vi "main.vi"() -> ()   [LabVIEW 2016]
uses:
  enum_setting_states.ctl
  <vilib>/Instr/_visa.llb/VISA Configure Serial Port (Instr).vi
  global.vi
panel:
  out "Tab Control":enum32{"Settings", "Data"}(tab)
  in  "Boolean":bool
  in  "4th":dbl=4.0 min=1.0 step=1.0 format="%#_3g"
  in  "3rd":dbl=3.0 min=1.0 step=1.0 format="%#_3g"
  in  "2nd":dbl=2.0 min=1.0 step=1.0 format="%#_3g"
  in  "1st":dbl=1.0 min=1.0 step=1.0 format="%#_3g"
  in  "START":bool
  in  "SET":bool
  in  "Flow control (None)":u16(ring) items=["None", "XON/XOFF", "RTS/CTS", "XON/XOFF & RTS/CTS", "DTR/DSR", "XON/XOFF & DTR/DSR"]
  in  "Parity (None)":enum16{"None", "Odd", "Even", "Mark", "Space"}(ring)
  in  "Stop bits (1)":u16(ring)=10 items=["1.0"=10, "1.5"=15, "2.0"=20]
  in  "Data bits (8)":u16=8 min=5 max=8 step=1
  in  "Baud rate (57600)":u32=57600
  in  "VISA resource name":refnum<visa-resource-name>="COM5"
  out "read buffer":string
  in  "Charge current":enum8{"0.25C", "0.5C", "1C"}(ring)=enum."0.5C"
  in  "Discharge current":enum8{"0.25C", "0.5C", "1C"}(ring)=enum."1C"
  in  "Number of cells":enum8{"", "1", "2", "3", "4"}(ring)=enum."1"
  in  "Options":T1(ring)=enum."Predischarge->Charge->Discharge->Postcharge"
  in  "Project Name":string="Test"
  out "Cell number":string
  out "State":string
  out "Path":path
  in  "stop":bool
  out "TEMP":dbl caption="Current Temperature\n(Celsius)"
  out "CURRENT":dbl caption="Current Temperature\n(Celsius)"
  out "VOLTAGE":dbl caption="Current Temperature\n(Celsius)"
  in  "next":bool
  out "Countdown":dbl caption="Current Temperature\n(Celsius)"
  out "min":dbl caption="Current Temperature\n(Celsius)"
  out "sec":dbl caption="Current Temperature\n(Celsius)"
  out "CAPACITY":dbl caption="Current Temperature\n(Celsius)"
  out "Voltage":cluster{dbl[], dbl[]}(graph)
  out "Current":cluster{dbl[], dbl[]}(graph)
  out "Temperature":cluster{dbl[], dbl[]}(graph)
  out "Capacity":cluster{dbl[], dbl[]}(graph)
  out "Received data":string
  # "UART configurations"
  # "Test configurations"
  # "Cell order"
  # "Elapsed time"
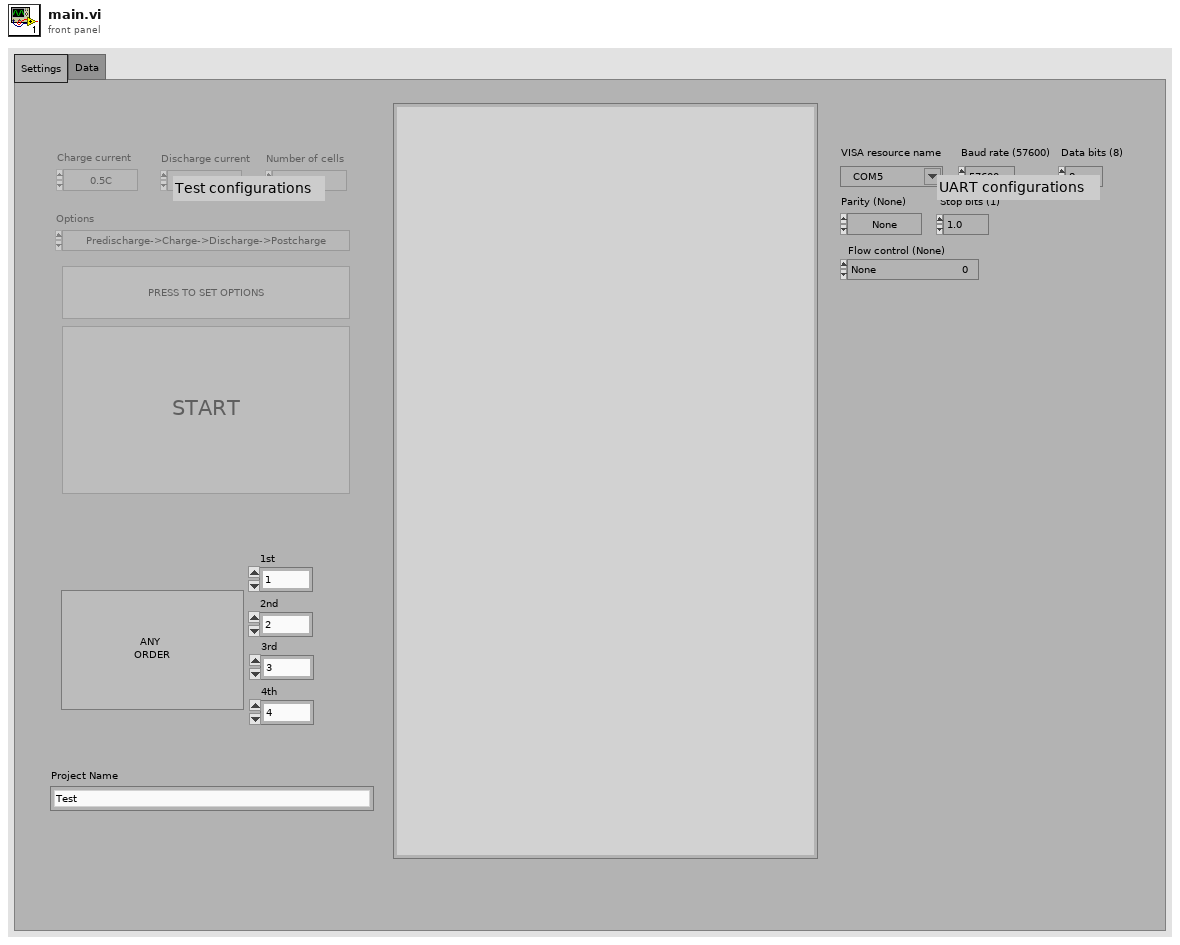
[diagram p1: front panel]
types:
  T1 = enum8{"", "Predischarge->Charge->Discharge->Postcharge", "Charge->Discharge", "Only Charge", "Only Discharge"}
  T2 = enum8{"Enabled", "Disabled", "Disabled and Grayed Out"}
  T3 = typedef "enum_setting_states.ctl" = enum16{"Initialize", "Charge_current", "Discharge_current", "Option", "Num_of_cells", "Start"}
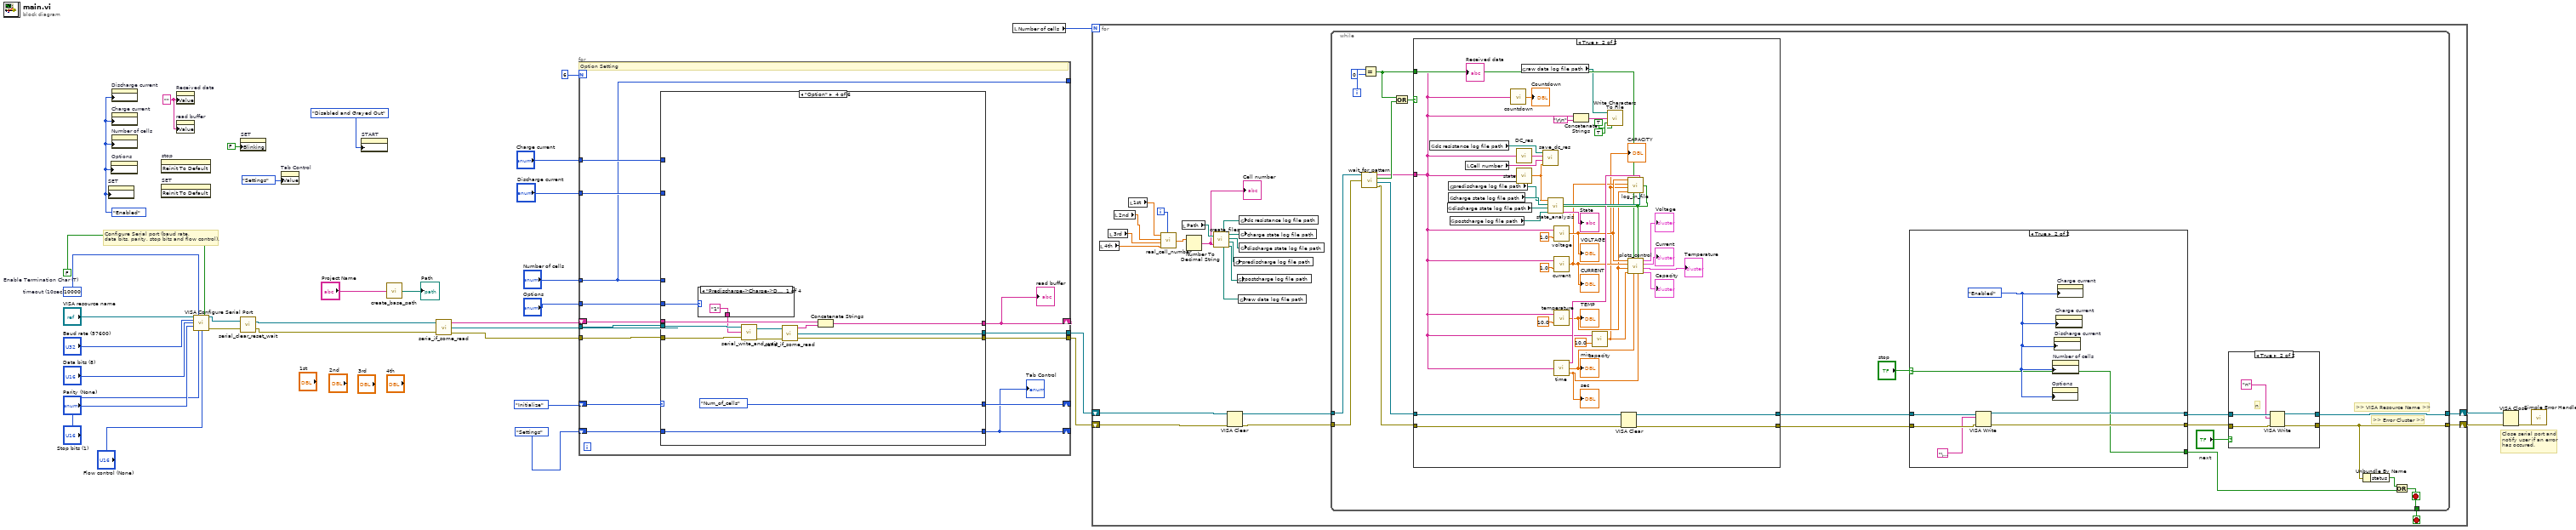
[diagram p0: block diagram]
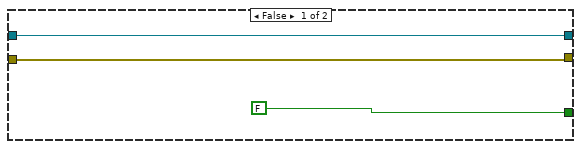
[diagram p4: hidden frame]
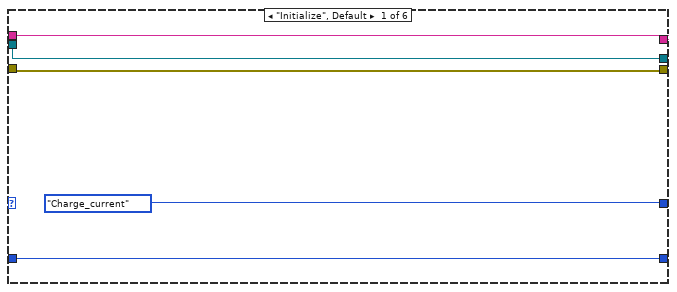
[diagram p5: hidden frame]
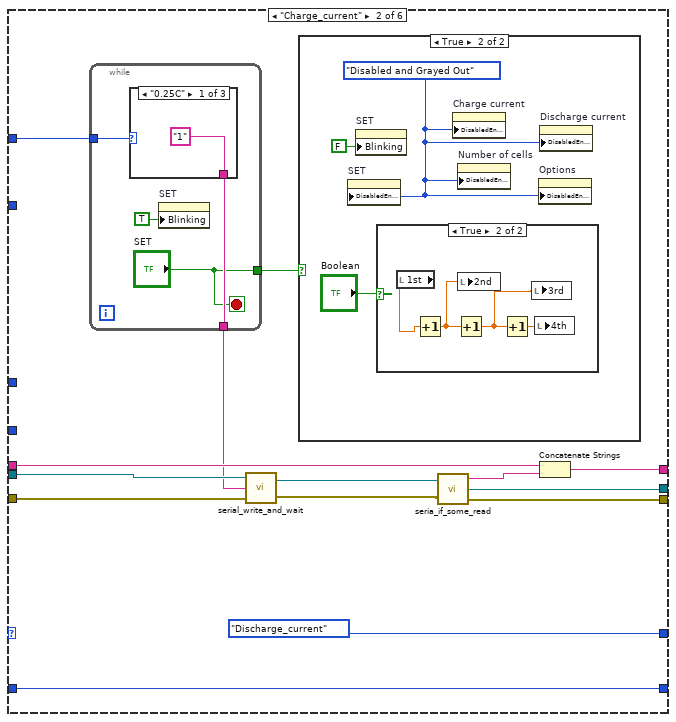
[diagram p6: hidden frame]
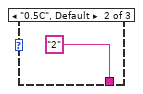
[diagram p9: hidden frame]
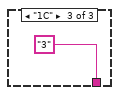
[diagram p10: hidden frame]
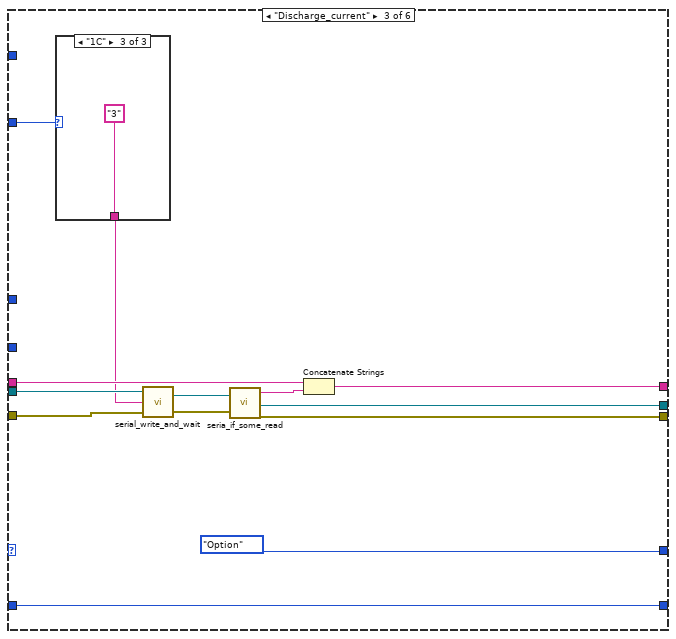
[diagram p11: hidden frame]
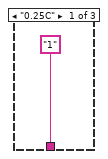
[diagram p12: hidden frame]
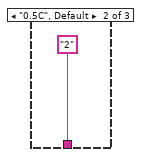
[diagram p13: hidden frame]
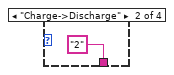
[diagram p14: hidden frame]
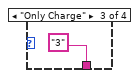
[diagram p15: hidden frame]
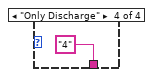
[diagram p16: hidden frame]
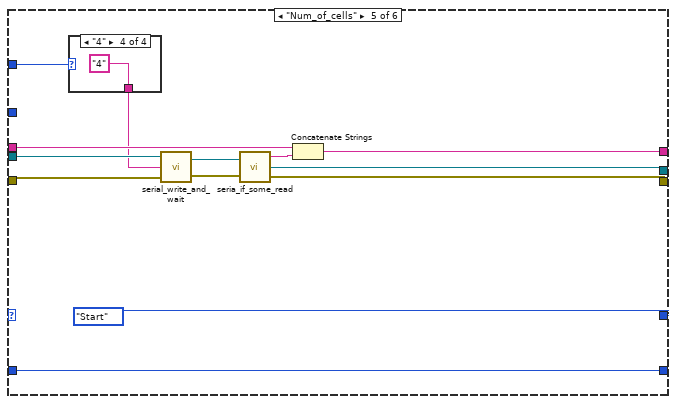
[diagram p17: hidden frame]
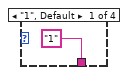
[diagram p18: hidden frame]
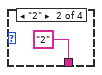
[diagram p19: hidden frame]
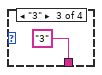
[diagram p20: hidden frame]
diagram:
  w12 = T2."Enabled" ("Disabled")
  w10 = "" ("read buffer")
  w34 = FALSE  # Enable Termination Char (T)
  w35 = u32 10000  # timeout (10sec)
  # "Close serial port and\nnotify user if an error\nhas occured."
  # "Configure Serial port (baud rate,\ndata bits, parity, stop bits and flow control)."
  n1 = property on="SET" class="Bool (strict)"("DisabledEnum"=w12) -> ()  [unwired: 2 in, 2 out]
  n2 = property on="Options" class="Enum (strict)"("DisabledEnum"=w12) -> ()  [unwired: 2 in, 2 out]
  n3 = property on="Discharge current" class="Enum (strict)"("DisabledEnum"=w12) -> ()  [unwired: 2 in, 2 out]
  n4 = property on="Charge current" class="Enum (strict)"("DisabledEnum"=w12) -> ()  [unwired: 2 in, 2 out]
  n5 = property on="Number of cells" class="Enum (strict)"("DisabledEnum"=w12) -> ()  [unwired: 2 in, 2 out]
  n6 = invoke on="stop" class="Bool" method="Reinit To Default"() -> ()  [unwired: 3 in, 3 out]
  n7 = invoke on="SET" class="Bool (strict)" method="Reinit To Default"() -> ()  [unwired: 3 in, 3 out]
  n8 = property on="Received data" class="Str"("Value"=w10) -> ()  [unwired: 2 in, 2 out]
  n9 = property on="read buffer" class="Str"("Value"=w10) -> ()  [unwired: 2 in, 2 out]
  n10 = call-poly "VISA Configure Serial Port"("VISA resource name"="VISA resource name", "timeout (10sec)"=w35, "Enable Termination\nChar (T)"=w34, "baud rate (9600)"="Baud rate (57600)", "data bits (8)"="Data bits (8)", "parity (0:none)"="Parity (None)", "stop bits (10: 1 bit)"="Stop bits (1)", "flow control (0:none)"="Flow control (None)") -> ("VISA resource name out"=w32:refnum<visa-resource-name>, "error out"=w33:errorcluster)  [unwired: 6 in]
  n11 = property on="SET" class="Bool (strict)"("Blinking"=FALSE) -> ()  [unwired: 2 in, 2 out]
  n12 = call "serial_clear_reset_wait.vi"("error in (no error)"=w33, "VISA Refnum in"=w32) -> ("error out"=w17:errorcluster, "VISA Refnum out"=w18:refnum<visa-resource-name>)
  n13 = property on="Tab Control" class="TabCtl (strict)"("Value"=enum32{"Settings", "Data"}."Settings" ("Tab Control")) -> ()  [unwired: 2 in, 2 out]
  n14 = property on="START" class="Bool"("DisabledEnum"=T2."Disabled and Grayed Out" ("Disabled")) -> ()  [unwired: 2 in, 2 out]
  n15 = call "create_base_path.vi"("project name"="Project Name") -> ("base path"=→"Path":path)
  n16 = call "seria_if_some_read.vi"("serial in"=w18, "error in (no error)"=w17) -> ("read buffer"=w8:string, "serial out"=w9:refnum<visa-resource-name>, "error out"=w20:errorcluster)
  n17 = for {
    N: 6 -> [_]
    shift-right: [w38] -> _
    shift-left: enum32{"Settings", "Data"}."Settings" ("Tab Control") -> [w47]
    shift-right: [w46] -> _
    shift-left: enum_setting_states."Initialize" -> [w45]
    tunnel: w9 -> [w43]
    tunnel: [w49] -> w3
    tunnel: w20 -> [w42]
    tunnel: [w48] -> w2
    tunnel: "Charge current" -> [w41]
    shift-right: [w44] -> _
    shift-left: w8 -> [w40]
    tunnel: "Discharge current" -> [w39]
    tunnel: "Number of cells" -> [w36]
    tunnel: "Options" -> [w37]
    tunnel: [w36] -> _
    # "Option Setting"
    n18 = case shown="\"Option\"" w45 {
      tunnel: w43 -> [w53 w66 w90 w103 w123 w140]
      tunnel: w42 -> [w52 w65 w88 w101 w121 w139]
      tunnel: [w51 w63 w93 w110 w126 w145] -> w44
      tunnel: [w53 w56 w84 w105 w117 w134] -> w49
      tunnel: [w52 w55 w83 w104 w116 w133] -> w48
      tunnel: [w50 w60 w91 w107 w124 enum32{"Settings", "Data"}."Data" ("Tab Control")] -> w38
      tunnel: w47 -> [w50 w60 w91 w107 w124 _]
      tunnel: [enum_setting_states."Charge_current" enum_setting_states."Discharge_current" enum_setting_states."Option" enum_setting_states."Num_of_cells" enum_setting_states."Start" enum_setting_states."Start"] -> w46
      tunnel: w40 -> [w51 w64 w94 w111 w127 w144]
      tunnel: w41 -> [_ w67 _ _ _ _]
      tunnel: w39 -> [_ _ w92 _ _ _]
      tunnel: w36 -> [_ _ _ _ w125 _]
      tunnel: w37 -> [_ _ _ w108 _ _]
      frame "Initialize", Default {
      }
      frame "Charge_current" {
        n19 = while {
          tunnel: w67 -> [w79]
          tunnel: [w78] -> w62
          tunnel: ["SET"] -> w61
          stop <- "SET" stop-if-true
          n20 = case shown="\"0.25C\"" w79 {
            tunnel: ["1" ("write buffer") "2" ("write buffer") "3" ("write buffer")] -> w78
            frame "0.25C" {
            }
            frame "0.5C", Default {
            }
            frame "1C" {
            }
          }
          n21 = property on="SET" class="Bool (strict)"("Blinking"=TRUE) -> ()  [unwired: 2 in, 2 out]
        }
        n22 = call "serial_write_and_wait.vi"("error in (no error)"=w65, "write buffer"=w62, "serial in"=w66) -> ("error out"=w58:errorcluster, "serial out"=w59:refnum<visa-resource-name>)
        n23 = case shown="True" w61 {
          frame False {
          }
          frame True {
            w70 = T2."Disabled and Grayed Out" ("Disabled")
            n24 = property on="SET" class="Bool (strict)"("DisabledEnum"=w70) -> ()  [unwired: 2 in, 2 out]
            n25 = property on="SET" class="Bool (strict)"("Blinking"=FALSE) -> ()  [unwired: 2 in, 2 out]
            n26 = case shown="True" "Boolean" {
              frame False {
              }
              frame True {
                n27 = local read "1st"() -> (w74:dbl)
                n28 = Increment(x=w74) -> (x+1=w75:dbl)
                n29 = Increment(x=w75) -> (x+1=w72:dbl)
                n30 = local write "2nd"(w75) -> ()
                n31 = Increment(x=w72) -> (x+1=w73:dbl)
                n32 = local write "3rd"(w72) -> ()
                n33 = local write "4th"(w73) -> ()
              }
            }
            n34 = property on="Charge current" class="Enum (strict)"("DisabledEnum"=w70) -> ()  [unwired: 2 in, 2 out]
            n35 = property on="Number of cells" class="Enum (strict)"("DisabledEnum"=w70) -> ()  [unwired: 2 in, 2 out]
            n36 = property on="Options" class="Enum (strict)"("DisabledEnum"=w70) -> ()  [unwired: 2 in, 2 out]
            n37 = property on="Discharge current" class="Enum (strict)"("DisabledEnum"=w70) -> ()  [unwired: 2 in, 2 out]
          }
        }
        n38 = call "seria_if_some_read.vi"("serial in"=w59, "error in (no error)"=w58) -> ("read buffer"=w57:string, "serial out"=w56:refnum<visa-resource-name>, "error out"=w55:errorcluster)
        n39 = Concatenate Strings(w64, w57) -> (w63:string)
      }
      frame "Discharge_current" {
        n40 = case shown="\"1C\"" w92 {
          tunnel: ["1" ("write buffer") "2" ("write buffer") "3" ("write buffer")] -> w89
          frame "0.25C" {
          }
          frame "0.5C", Default {
          }
          frame "1C" {
          }
        }
        n41 = call "serial_write_and_wait.vi"("error in (no error)"=w88, "write buffer"=w89, "serial in"=w90) -> ("error out"=w86:errorcluster, "serial out"=w87:refnum<visa-resource-name>)
        n42 = call "seria_if_some_read.vi"("serial in"=w87, "error in (no error)"=w86) -> ("read buffer"=w85:string, "serial out"=w84:refnum<visa-resource-name>, "error out"=w83:errorcluster)
        n43 = Concatenate Strings(w94, w85) -> (w93:string)
      }
      frame "Option" {
        n44 = case shown="\"Predischarge->Charge->Discharge->Postcharge\", Default" w108 {
          tunnel: ["1" ("write buffer") "2" ("write buffer") "3" ("write buffer") "4" ("write buffer")] -> w102
          frame "Predischarge->Charge->Discharge->Postcharge", Default {
          }
          frame "Charge->Discharge" {
          }
          frame "Only Charge" {
          }
          frame "Only Discharge" {
          }
        }
        n45 = call "serial_write_and_wait.vi"("error in (no error)"=w101, "write buffer"=w102, "serial in"=w103) -> ("error out"=w99:errorcluster, "serial out"=w100:refnum<visa-resource-name>)
        n46 = call "seria_if_some_read.vi"("serial in"=w100, "error in (no error)"=w99) -> ("read buffer"=w106:string, "serial out"=w105:refnum<visa-resource-name>, "error out"=w104:errorcluster)
        n47 = Concatenate Strings(w111, w106) -> (w110:string)
      }
      frame "Num_of_cells" {
        n48 = case shown="\"4\"" w125 {
          tunnel: ["1" ("write buffer") "2" ("write buffer") "3" ("write buffer") "4" ("write buffer")] -> w122
          frame "1", Default {
          }
          frame "2" {
          }
          frame "3" {
          }
          frame "4" {
          }
        }
        n49 = call "serial_write_and_wait.vi"("error in (no error)"=w121, "write buffer"=w122, "serial in"=w123) -> ("error out"=w119:errorcluster, "serial out"=w120:refnum<visa-resource-name>)
        n50 = call "seria_if_some_read.vi"("serial in"=w120, "error in (no error)"=w119) -> ("read buffer"=w118:string, "serial out"=w117:refnum<visa-resource-name>, "error out"=w116:errorcluster)
        n51 = Concatenate Strings(w127, w118) -> (w126:string)
      }
      frame "Start" {
        n52 = while {
          tunnel: ["s" ("write buffer")] -> w138
          tunnel: ["START"] -> w141
          stop <- "START" stop-if-true
          n53 = property on="START" class="Bool"("DisabledEnum"=T2."Enabled" ("Disabled")) -> ()  [unwired: 2 in, 2 out]
        }
        n54 = case shown="True" w141 {
          frame False {
          }
          frame True {
            n55 = property on="START" class="Bool"("DisabledEnum"=T2."Disabled and Grayed Out" ("Disabled")) -> ()  [unwired: 2 in, 2 out]
          }
        }
        n56 = call "serial_write_and_wait.vi"("error in (no error)"=w139, "write buffer"=w138, "serial in"=w140) -> ("error out"=w136:errorcluster, "serial out"=w137:refnum<visa-resource-name>)
        n57 = call "seria_if_some_read.vi"("serial in"=w137, "error in (no error)"=w136) -> ("read buffer"=w135:string, "serial out"=w134:refnum<visa-resource-name>, "error out"=w133:errorcluster)
        n58 = Concatenate Strings(w144, w135) -> (w145:string)
      }
    }
    "read buffer" <- w44
    "Tab Control" <- w38
  }
  n59 = local read "Number of cells"() -> (w1:enum8{"", "1", "2", "3", "4"})
  n60 = for {
    N: w1 -> [_]
    shift-right: [w168] -> w24
    shift-left: w3 -> [w166]
    shift-right: [w167] -> w23
    shift-left: w2 -> [w165]
    i -> [w152]
    stop <- w164 stop-if-true
    n61 = local read "4th"() -> (w163:dbl)
    n62 = local read "3rd"() -> (w162:dbl)
    n63 = local read "2nd"() -> (w161:dbl)
    n64 = local read "1st"() -> (w160:dbl)
    n65 = call "real_cell_number.vi"("1st"=w160, "2nd"=w161, "3rd"=w162, "4th"=w163, "current loop (cell)"=w152) -> ("real cell number"=w159:dbl)
    n66 = local read "Path"() -> (w158:path)
    n67 = Number To Decimal String(number=w159) -> (decimal integer string=w153:string)  [unwired: 1 in]
    "Cell number" <- w153
    n68 = call "create_files.vi"("base path"=w158, "cell number string"=w153) -> ("dc resistance log file path"=w154:path, "raw data log file path"=w157:path, "charge state log file path"=w156:path, "discharge state log file path"=w155:path, "predischarge state log file path"=w151:path, "postcharge state log file path"=w150:path)
    n69 = VISA Clear(VISA resource name=w166, error in (no error)=w165) -> (VISA resource name out=w170:refnum<visa-resource-name>, error out=w169:errorcluster)
    n70 = global write "global.vi" "predischarge log file path"(w151) -> ()
    n71 = global write "global.vi" "postcharge log file path"(w150) -> ()
    n72 = global write "global.vi" "raw data log file path"(w157) -> ()
    n73 = global write "global.vi" "dc resistance log file path"(w154) -> ()
    n74 = global write "global.vi" "charge state log file path"(w156) -> ()
    n75 = global write "global.vi" "discharge state log file path"(w155) -> ()
    n76 = while {
      tunnel: [w188] -> w168
      tunnel: w170 -> [w178]
      tunnel: w169 -> [w177]
      tunnel: [w187] -> w167
      tunnel: [w186] -> w164
      i -> [w183]
      stop <- w186 stop-if-true
      # ">> Error Cluster >>"
      # ">> VISA Resource Name >>"
      n77 = call "wait_for_pattern.vi"("serial in"=w178, "error in (no error)"=w177) -> ("pattern string"=w173:string, "pattern detected"=w176:bool, "serial out"=w174:refnum<visa-resource-name>, "error out"=w175:errorcluster)  [unwired: 1 in]
      n78 = Equal?(x=w183, y=0) -> (x = y?=w180:bool)
      n79 = Or(x=w180, y=w176) -> (x .or. y?=w181:bool)
      n80 = case shown="True" w181 {
        tunnel: w173 -> [_ w195]
        tunnel: w174 -> [w193 w213]
        tunnel: w175 -> [w192 w211]
        tunnel: [w192 w210] -> w185
        tunnel: [w193 w212] -> w184
        tunnel: w180 -> [_ w202]
        frame False {
        }
        frame True {
          n81 = global read "global.vi" "dc resistance log file path"() -> (w198:path)
          n82 = global read "global.vi" "discharge state log file path"() -> (w200:path)
          n83 = global read "global.vi" "predischarge log file path"() -> (w199:path)
          n84 = global read "global.vi" "charge state log file path"() -> (w201:path)
          n85 = global read "global.vi" "postcharge log file path"() -> (w194:path)
          n86 = local read "Cell number"() -> (w196:string)
          n87 = call "countdown.vi"("buffer in"=w195) -> ("countdown"=→"Countdown":dbl)
          n88 = call "DC_res.vi"("read buffer in"=w195) -> ("read buffer out"=w224:string)
          n89 = call "state.vi"("buffer in"=w195) -> ("current state"=w223:dbl)
          n90 = global read "global.vi" "raw data log file path"() -> (w197:path)
          n91 = call "save_dc_res.vi"("current state"=w223, "cell number"=w196, "dc resistance"=w224, "file path"=w198) -> ()
          n92 = call "state_analysis.vi"("current state number"=w223, "postcharge state log file path"=w194, "discharge state log file path"=w200, "charge state log file path"=w201, "predischarge state log file path"=w199) -> ("current state name"=→"State":string, "log? plot?"=w209:bool, "chosen log file path"=w227:path)
          n93 = call "time.vi"("buffer in"=w195) -> ("mm:ss"=w222:string, "minutes"=w208:dbl, "seconds"=w207:dbl)
          "min" <- w208
          "sec" <- w207
          n94 = call "voltage.vi"("divider"=1.0 ("y"), "buffer in"=w195) -> ("voltage"=w206:dbl)
          "VOLTAGE" <- w206
          n95 = call "current.vi"("divider"=1.0 ("y"), "buffer in"=w195) -> ("current"=w205:dbl)
          "CURRENT" <- w205
          n96 = call "temperature.vi"("divider"=10.0 ("y"), "buffer in"=w195) -> ("temperature"=w204:dbl)
          "TEMP" <- w204
          n97 = Concatenate Strings(w195, "\r\n") -> (w217:string)
          n98 = call "capacity.vi"("divider"=10.0 ("y"), "buffer in"=w195) -> ("capacity"=w203:dbl)
          "CAPACITY" <- w203
          n99 = call <vilib>:"Write Characters To File.vi"("convert eol? (no:F)"=TRUE, "append to file? (new file:F)"=TRUE, "character string"=w217, "file path (dialog if empty)"=w197) -> ()  [unwired: 1 in, 1 out]
          n100 = VISA Clear(VISA resource name=w213, error in (no error)=w211) -> (VISA resource name out=w212:refnum<visa-resource-name>, error out=w210:errorcluster)
          n101 = call "log_in_file.vi"("file path"=w227, "save?"=w209, "mm:ss"=w222, "temperature"=w204, "capacity"=w203, "current"=w205, "voltage"=w206) -> ()
          n102 = call "plots_control.vi"("seconds"=w207, "log? plot?"=w209, "minutes"=w208, "is first loop?"=w202, "capacity"=w203, "temperature"=w204, "current"=w205, "voltage"=w206) -> ("capacity cluster"=→"Capacity":cluster{dbl[], dbl[]}, "temperature cluster"=→"Temperature":cluster{dbl[], dbl[]}, "current cluster"=→"Current":cluster{dbl[], dbl[]}, "voltage cluster"=→"Voltage":cluster{dbl[], dbl[]})
          "Received data" <- w195
        }
      }
      n103 = case shown="True" "stop" {
        selector: "stop" -> [_ w242]
        tunnel: w184 -> [w240 w248]
        tunnel: [w240 w247] -> w190
        tunnel: w185 -> [w241 w246]
        tunnel: [w241 w245] -> w189
        tunnel: [FALSE w242] -> w172
        frame False {
        }
        frame True {
          w243 = T2."Enabled" ("Disabled")
          n104 = VISA Write(VISA resource name=w248, write buffer="\u001b", error in (no error)=w246) -> (VISA resource name out=w247:refnum<visa-resource-name>, error out=w245:errorcluster)  [unwired: 1 out]
          n105 = property on="Options" class="Enum (strict)"("DisabledEnum"=w243) -> ()  [unwired: 2 in, 2 out]
          n106 = property on="Number of cells" class="Enum (strict)"("DisabledEnum"=w243) -> ()  [unwired: 2 in, 2 out]
          n107 = property on="Discharge current" class="Enum (strict)"("DisabledEnum"=w243) -> ()  [unwired: 2 in, 2 out]
          n108 = property on="Charge current" class="Enum (strict)"("DisabledEnum"=w243) -> ()  [unwired: 2 in, 2 out]
          n109 = property on="Charge current" class="Enum (strict)"("DisabledEnum"=w243) -> ()  [unwired: 2 in, 2 out]
        }
      }
      n110 = case shown="True" "next" {
        tunnel: w190 -> [w232 w238]
        tunnel: [w232 w237] -> w188
        tunnel: w189 -> [w233 w236]
        tunnel: [w233 w235] -> w187
        frame False {
        }
        frame True {
          # "n"
          n111 = VISA Write(VISA resource name=w238, write buffer="n", error in (no error)=w236) -> (VISA resource name out=w237:refnum<visa-resource-name>, error out=w235:errorcluster)  [unwired: 1 out]
        }
      }
      n112 = Unbundle By Name(w187) -> ("status"=w171:bool)
      n113 = Or(x=w171, y=w172) -> (x .or. y?=w186:bool)
    }
  }
  n114 = VISA Close(VISA resource name=w24, error in (no error)=w23) -> (error out=w25:errorcluster)
  n115 = call <vilib>:"Simple Error Handler.vi"("error in (no error)"=w25) -> ()  [unwired: 4 in, 5 out]
